vi "华为UPS2000-G通信.vi"() -> ()   [LabVIEW 2016, in "环境动力监测库.lvlib" / "UPS库.lvlib"]
panel:
  out "UPS参数":T1 {"开机状态" items=["关机", "开机中", "开机失败", "开机完成"]}
  in  "开机":bool
  out "UPS状态":bool[](array[boolean])
  out "电池状态":T2 {"电池状态" items=["休眠"=2, "浮充"=3, "均充"=4, "放电"=5]}
  in  "open":bool
  in  "close":bool
  out "通信指示":bool
  in  "关机":bool
  in  "状态查询":bool
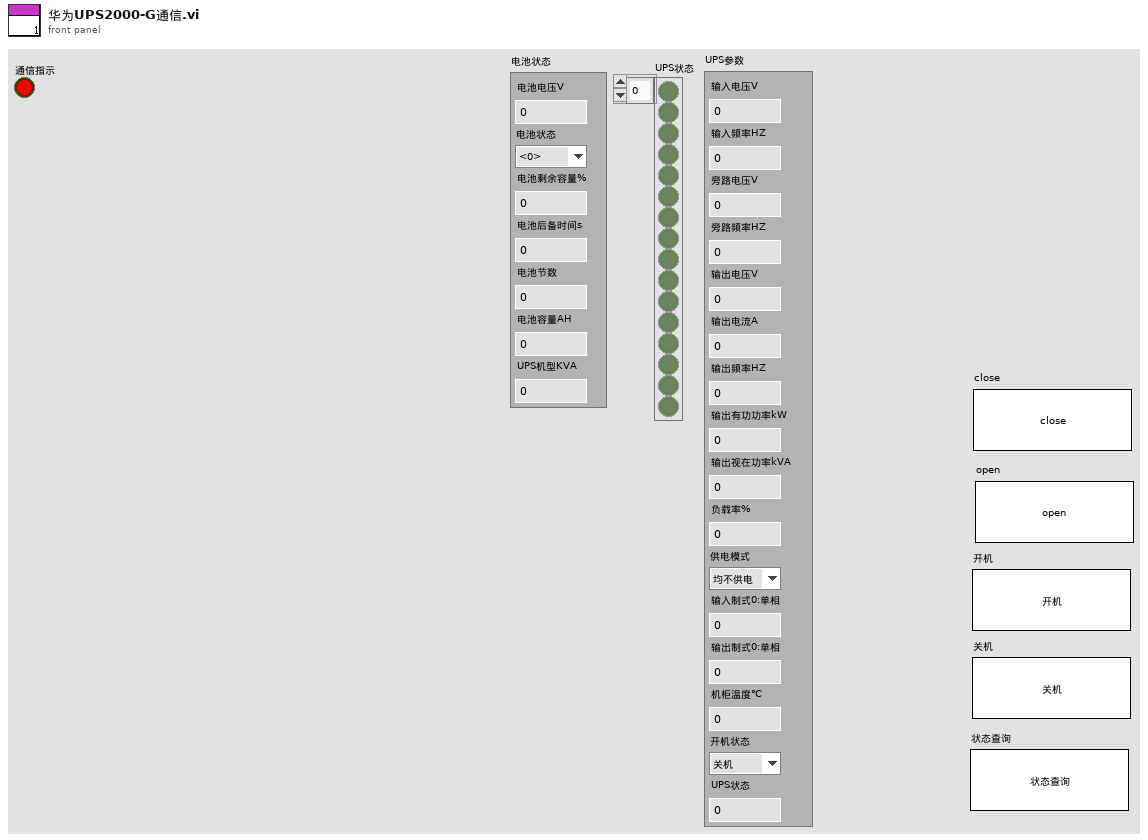
[diagram p1: front panel]
types:
  T1 = cluster{"输入电压V":dbl, "输入频率HZ":dbl, "旁路电压V":dbl, "旁路频率HZ":dbl, "输出电压V":dbl, "输出电流A":dbl, "输出频率HZ":dbl, "输出有功功率kW":dbl, "输出视在功率kVA":dbl, "负载率%":dbl, "供电模式":enum16{"均不供电", "旁路供电", "主路供电", "电池供电", "主路ECO"}, "输入制式0:单相":u16, "输出制式0:单相":u16, "机柜温度℃":dbl, "开机状态":u16, "UPS状态":u8}
  T2 = cluster{"电池电压V":dbl, "电池状态":u16, "电池剩余容量%":u16, "电池后备时间s":u32, "电池节数":u16, "电池容量AH":u16, "UPS机型KVA":u16}
  T3 = cluster{"VISA resource name":refnum<visa-resource-name>, "Serial Config":cluster{"baud rate (9600)":u32, "stop bits (10: 1 bit)":u16, "parity (0:none)":enum16{"None", "Odd", "Even", "Mark", "Space"}, "data bits (8)":u16, "timeout (10sec)":u32}, "型号选择":enum16{"山特UPSC1~3", "山特UPSC6~20", "华为UPS2000-G-(1-3KVA)"}, "HW-UPS-2000 MB session":refnum<class "MB_Master.lvclass">, "连接方式":enum16{"串口", "TCP"}, "IP":string, "Port":string}
  T4 = cluster{"baud rate (bps)":u32, "stop bits":u16, "parity":u16, "flow control":u16, "timeout":u32, "retries":i32}
  T5 = cluster{"baud rate (9600)":u32, "stop bits (10: 1 bit)":u16, "parity (0:none)":enum16{"None", "Odd", "Even", "Mark", "Space"}, "data bits (8)":u16, "timeout (10sec)":u32}
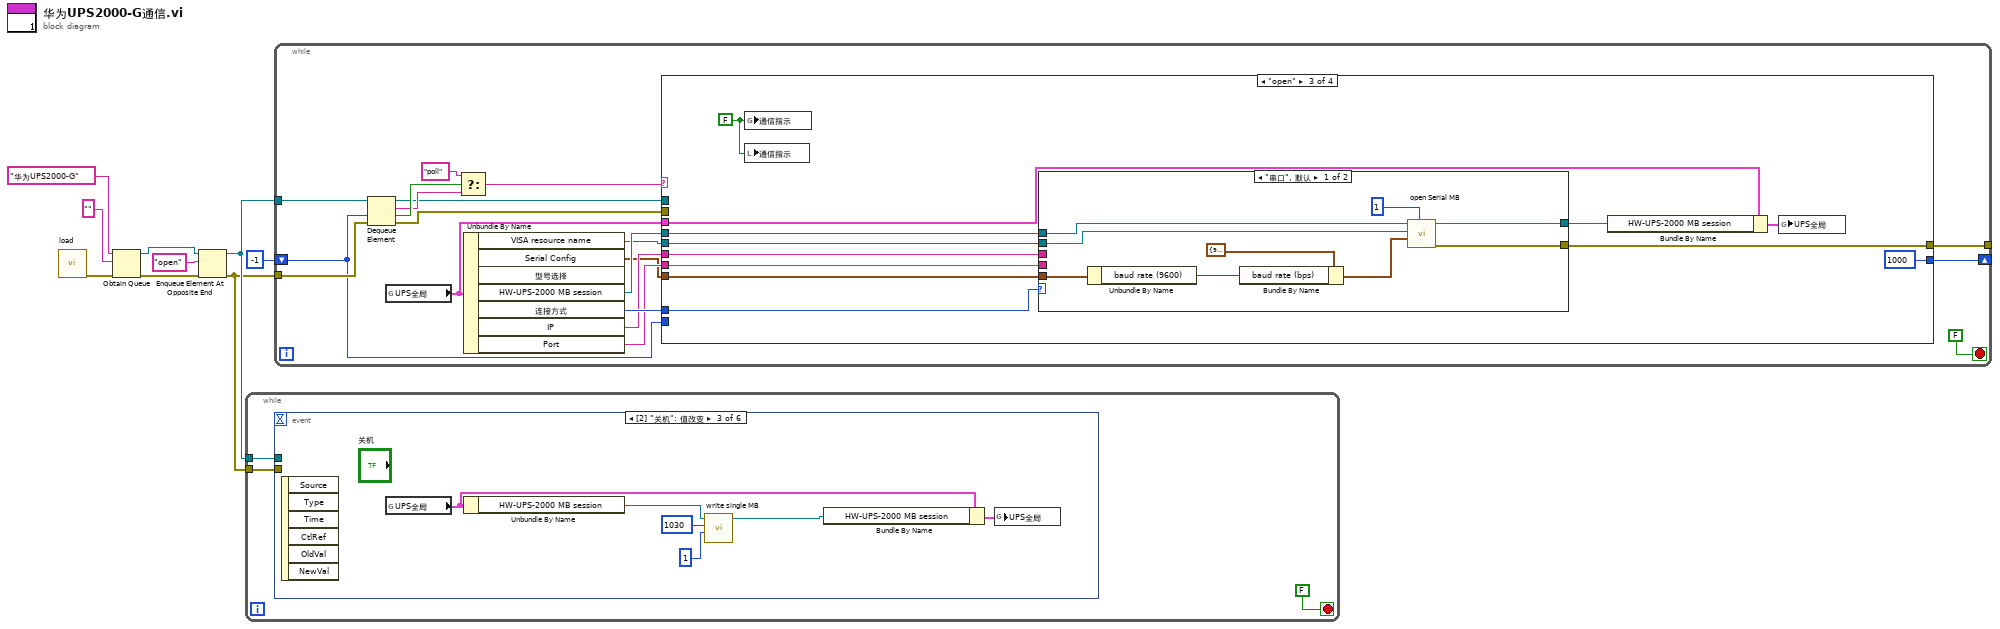
[diagram p0: block diagram]
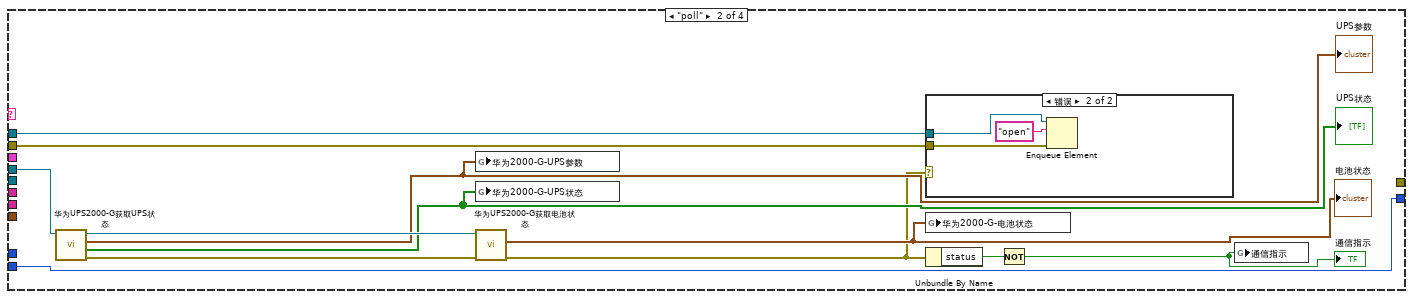
[diagram p3: hidden frame]
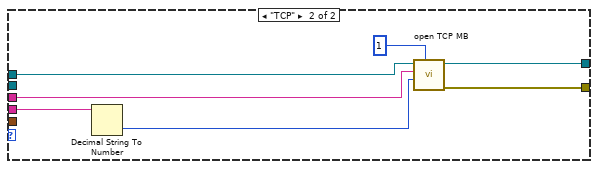
[diagram p5: hidden frame]
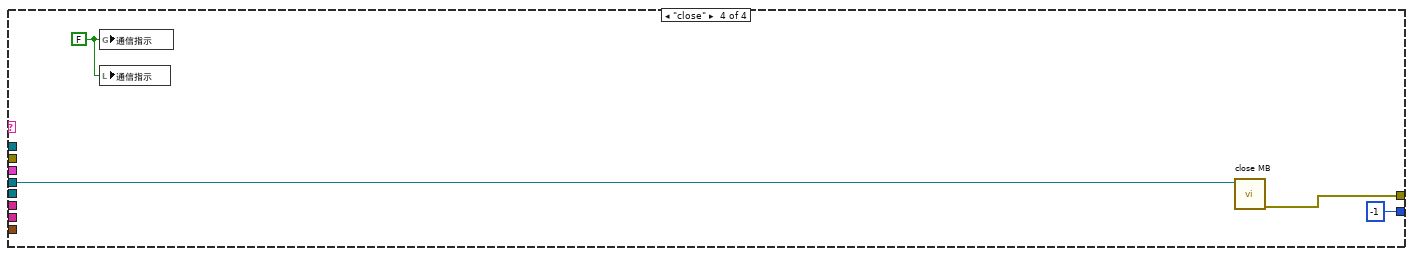
[diagram p6: hidden frame]
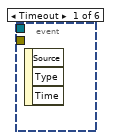
[diagram p7: hidden frame]
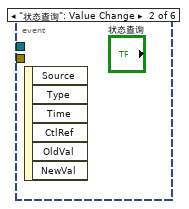
[diagram p8: hidden frame]
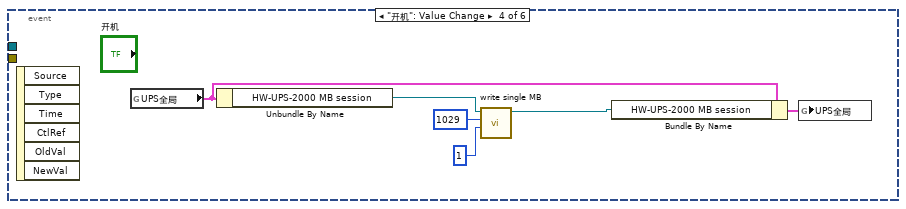
[diagram p9: hidden frame]
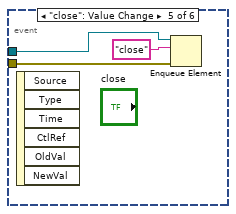
[diagram p10: hidden frame]
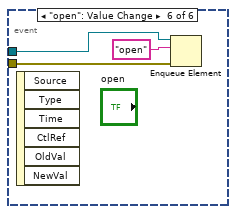
[diagram p11: hidden frame]
diagram:
  n1 = call "load.vi"() -> ("error out"=w1:errorcluster)  [unwired: 11 in]
  n2 = Obtain Queue(name (unnamed)="华为UPS2000-G" ("名称（未命名）"), element data type="", error in (no error)=w1) -> (queue out=w6:refnum<queue>, error out=w5:errorcluster)  [unwired: 2 in, 1 out]
  n3 = Enqueue Element At Opposite End(queue=w6, element="open" ("元素"), error in (no error)=w5) -> (queue out=w3:refnum<queue>, error out=w2:errorcluster)  [unwired: 1 in, 1 out]
  n4 = while {
    tunnel: w3 -> [w11]
    tunnel: w2 -> [w10]
    stop <- FALSE stop-if-true
    n5 = event shown="[2] \"关机\": 值改变" {
      selector: _ -> [_ _ _ _ _ _]
      dyn-events: _ -> [_ _ _ _ _ _]
      timeout: _ -> [_ _ _ _ _ _]
      tunnel: w11 -> [_ _ _ _ w26 w29]
      tunnel: w10 -> [_ _ _ _ w25 w28]
      event Timeout {
        n6 = event-data() -> ()  [unwired: 1 in, 3 out]
      }
      event "状态查询": Value Change {
        n7 = event-data() -> ()  [unwired: 1 in, 6 out]
      }
      event "关机": Value Change {
        n8 = event-data() -> ()  [unwired: 1 in, 6 out]
        n9 = global read "断电保存全局变量.vi" "UPS全局"() -> (w13:T3)
        n10 = Unbundle By Name(w13) -> ("HW-UPS-2000 MB session"=w16:refnum<class "MB_Master.lvclass">)
        n11 = call "write single MB.vi"("value"=u16 1, "address"=u16 1030, "MB session in"=w16) -> ("MB session out"=w14:refnum<class "MB_Master.lvclass">)  [unwired: 7 in, 1 out]
        n12 = Bundle By Name(cluster=w13, "HW-UPS-2000 MB session"=w14) -> (w15:T3)
        n13 = global write "断电保存全局变量.vi" "UPS全局"(w15) -> ()
      }
      event "开机": Value Change {
        n14 = event-data() -> ()  [unwired: 1 in, 6 out]
        n15 = global read "断电保存全局变量.vi" "UPS全局"() -> (w19:T3)
        n16 = Unbundle By Name(w19) -> ("HW-UPS-2000 MB session"=w22:refnum<class "MB_Master.lvclass">)
        n17 = call "write single MB.vi"("value"=u16 1, "address"=u16 1029, "MB session in"=w22) -> ("MB session out"=w20:refnum<class "MB_Master.lvclass">)  [unwired: 7 in, 1 out]
        n18 = Bundle By Name(cluster=w19, "HW-UPS-2000 MB session"=w20) -> (w21:T3)
        n19 = global write "断电保存全局变量.vi" "UPS全局"(w21) -> ()
      }
      event "close": Value Change {
        n20 = event-data() -> ()  [unwired: 1 in, 6 out]
        n21 = Enqueue Element(queue=w26, element="close" ("元素"), error in (no error)=w25) -> ()  [unwired: 1 in, 3 out]
      }
      event "open": Value Change {
        n22 = event-data() -> ()  [unwired: 1 in, 6 out]
        n23 = Enqueue Element(queue=w29, element="open" ("元素"), error in (no error)=w28) -> ()  [unwired: 1 in, 3 out]
      }
    }
  }
  n24 = while {
    tunnel: w3 -> [w46]
    tunnel: w2 -> [w45]
    shift-right: [w42] -> _
    shift-left: -1 ("超时毫秒(-1)") -> [w43]
    tunnel: [w41] -> _
    stop <- FALSE stop-if-true
    n25 = Dequeue Element(queue=w46, timeout in ms (-1)=w43, error in (no error)=w45) -> (queue out=w39:refnum<queue>, element=w47:string, timed out?=w49:bool, error out=w38:errorcluster)
    n26 = global read "断电保存全局变量.vi" "UPS全局"() -> (w33:T3)
    n27 = Select(t="poll" ("元素"), s=w49, f=w47) -> (s? t:f=w44:string)
    n28 = Unbundle By Name(w33) -> ("VISA resource name"=w32:refnum<visa-resource-name>, "Serial Config"=w31:T5, "HW-UPS-2000 MB session"=w37:refnum<class "MB_Master.lvclass">, "连接方式"=w36:enum16{"串口", "TCP"}, "IP"=w35:string, "Port"=w34:string)  [unwired: 1 out]
    n29 = case shown="\"open\"" w44 {
      tunnel: w43 -> [w50 w62 _ _]
      tunnel: [w50 w62 1000 ("超时毫秒(-1)") -1 ("超时毫秒(-1)")] -> w42
      tunnel: w37 -> [_ w61 w77 w96]
      tunnel: [_ _ w75 w94] -> w41
      tunnel: w39 -> [_ w52 _ _]
      tunnel: w38 -> [_ w51 _ _]
      tunnel: w36 -> [_ _ w73 _]
      tunnel: w35 -> [_ _ w72 _]
      tunnel: w34 -> [_ _ w71 _]
      tunnel: w33 -> [_ _ w70 _]
      tunnel: w32 -> [_ _ w67 _]
      tunnel: w31 -> [_ _ w66 _]
      frame Default {
      }
      frame "poll" {
        n30 = call "华为UPS2000-G获取UPS状态.vi"("MB session in"=w61) -> ("error out"=w59:errorcluster, "UPS状态"=w56:bool[], "UPS参数"=w57:T1, "MB session out"=w60:refnum<class "MB_Master.lvclass">)  [unwired: 7 in]
        "UPS状态" <- w56
        "UPS参数" <- w57
        n31 = global write "UPS内部交互全局.vi" "华为2000-G-UPS参数"(w57) -> ()
        n32 = global write "UPS内部交互全局.vi" "华为2000-G-UPS状态"(w56) -> ()
        n33 = call "华为UPS2000-G获取电池状态.vi"("error in (no error)"=w59, "MB session in"=w60) -> ("error out"=w53:errorcluster, "电池状态"=w55:T2)  [unwired: 7 in, 1 out]
        "电池状态" <- w55
        n34 = case shown="错误" w53 {
          tunnel: w52 -> [_ w64]
          tunnel: w51 -> [_ w63]
          frame No Error {
          }
          frame Error {
            n35 = Enqueue Element(queue=w64, element="open" ("元素"), error in (no error)=w63) -> ()  [unwired: 1 in, 3 out]
          }
        }
        n36 = global write "UPS内部交互全局.vi" "华为2000-G-电池状态"(w55) -> ()
        n37 = Unbundle By Name(w53) -> ("status"=w58:bool)
        n38 = Not(x=w58) -> (.not. x?=w54:bool)
        "通信指示" <- w54
        n39 = global write "UPS内部交互全局.vi" "通信指示"(w54) -> ()
      }
      frame "open" {
        w74 = FALSE ("通讯状态 2")
        n40 = global write "UPS内部交互全局.vi" "通信指示"(w74) -> ()
        n41 = local write "通信指示"(w74) -> ()
        n42 = case shown="\"串口\", 默认" w73 {
          tunnel: [w82 w90] -> w69
          tunnel: w77 -> [w81 w93]
          tunnel: [w80 w89] -> w75
          tunnel: w72 -> [_ w88]
          tunnel: w71 -> [_ w87]
          tunnel: w67 -> [w79 _]
          tunnel: w66 -> [w78 _]
          frame "串口", Default {
            n43 = Unbundle By Name(w78) -> ("baud rate (9600)"=w84:u32)
            n44 = Bundle By Name(cluster=T4 {"baud rate (bps)"=9600, "stop bits"=10, "parity"=0, "flow control"=0, "timeout"=1000, "retries"=1} ("Serial Config"), "baud rate (bps)"=w84) -> (w83:T4)
            n45 = call "open Serial MB.vi"("Slave ID"=u8 1, "Serial Config"=w83, "VISA Resource"=w79, "MB session in"=w81) -> ("error out"=w80:errorcluster, "MB session out"=w82:refnum<class "MB_Master.lvclass">)  [unwired: 6 in]
          }
          frame "TCP" {
            n46 = Decimal String To Number(string=w87) -> (number=w92:i32)  [unwired: 2 in, 1 out]
            n47 = call "open TCP MB.vi"("Slave ID (255)"=u8 1 ("Slave ID"), "Port (502)"=w92, "IP Address"=w88, "MB session in"=w93) -> ("error out"=w89:errorcluster, "MB session out"=w90:refnum<class "MB_Master.lvclass">)  [unwired: 6 in]
          }
        }
        n48 = Bundle By Name(cluster=w70, "HW-UPS-2000 MB session"=w69) -> (w68:T3)
        n49 = global write "断电保存全局变量.vi" "UPS全局"(w68) -> ()
      }
      frame "close" {
        w97 = FALSE ("通讯状态 2")
        n50 = global write "UPS内部交互全局.vi" "通信指示"(w97) -> ()
        n51 = local write "通信指示"(w97) -> ()
        n52 = call "close MB.vi"("MB session in"=w96) -> ("error out"=w94:errorcluster)  [unwired: 10 in]
      }
    }
  }
